vi "Init.vi"(5 "Overwrite Lib Path":path, 7 "ndim":i32, 8 "error in (no error)":errorcluster, 9 "flann_params":T1={"algorithm"=0, "checks"=0, "eps"=0.0, "sorted"=1, "max_neighbors"=-1, "cores"=0, "trees"=0, "leaf_max_size"=0, "branching"=0, "iterations"=0, "centers_init"=0, "cb_index"=0.0, "target_precision"=0.0, "build_weight"=0.0, "memory_weight"=0.0, "sample_fraction"=0.0, "table_number_"=0, "key_size_"=0, "multi_probe_level_"=0, "log_level"=0, "random_seed"=0} {"algorithm" items=["FLANN_INDEX_LINEAR"=0, "FLANN_INDEX_KDTREE"=1, "FLANN_INDEX_KMEANS"=2, "FLANN_INDEX_COMPOSITE"=3, "FLANN_INDEX_KDTREE_SINGLE"=4, "FLANN_INDEX_HIERARCHICAL"=5, "FLANN_INDEX_LSH"=6, "FLANN_INDEX_SAVED"=254, "FLANN_INDEX_AUTOTUNED"=255]; "centers_init" items=["FLANN_CENTERS_RANDOM", "FLANN_CENTERS_GONZALES", "FLANN_CENTERS_KMEANSPP", "FLANN_CENTERS_GROUPWISE"]; "log_level" items=["FLANN_LOG_NONE", "FLANN_LOG_FATAL", "FLANN_LOG_ERROR", "FLANN_LOG_WARN", "FLANN_LOG_INFO", "FLANN_LOG_DEBUG"]}, 10 "index_ptr":u64, 11 "KD Tree in":refnum<class "KD Tree.lvclass">) -> (0 "error out":errorcluster, 3 "KD Tree out":refnum<class "KD Tree.lvclass">)   [LabVIEW 2020, in "KD Tree.lvlib" / "KD Tree.lvclass"]
uses:
  KD Tree.lvclass
  flann/Flann Params.ctl
  KD Tree.lvclass/KD Tree.ctl
  KD Tree.lvlib
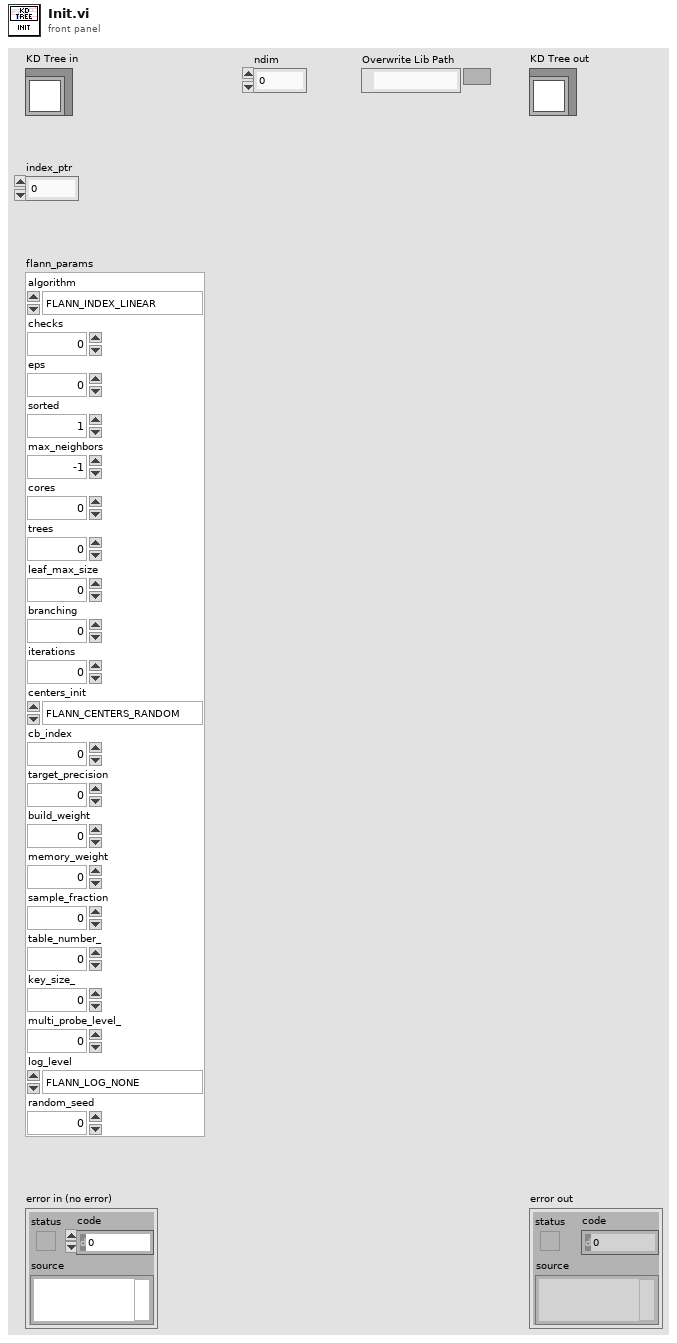
[diagram p1: front panel]
types:
  T1 = typedef "KD Tree.lvlib/Flann Params.ctl" = cluster{"algorithm":u32, "checks":i32, "eps":sgl, "sorted":i32, "max_neighbors":i32, "cores":i32, "trees":i32, "leaf_max_size":i32, "branching":i32, "iterations":i32, "centers_init":u32, "cb_index":sgl, "target_precision":sgl, "build_weight":sgl, "memory_weight":sgl, "sample_fraction":sgl, "table_number_":u32, "key_size_":u32, "multi_probe_level_":u32, "log_level":u32, "random_seed":i32}
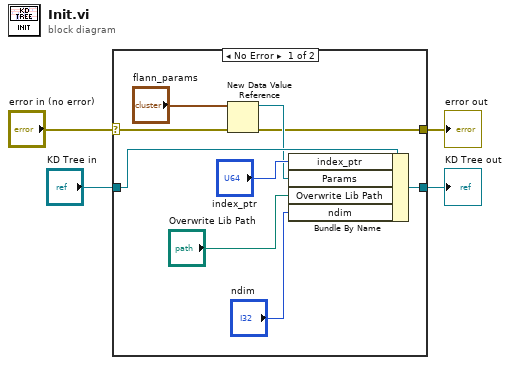
[diagram p0: block diagram]
diagram:
  n1 = case shown="No Error" "error in (no error)" {
    selector: "error in (no error)" -> [w12 w15]
    tunnel: [w5 w15] -> w3
    tunnel: [w11 w14] -> w1
    tunnel: "KD Tree in" -> [w13 w14]
    frame No Error {
      n2 = New Data Value Reference(data value="flann_params", error in=w12) -> (data value reference=w9:refnum<data-value>, error out=w5:errorcluster)
      n3 = Bundle By Name(cluster=w13, "index_ptr"="index_ptr", "Params"=w9, "Overwrite Lib Path"="Overwrite Lib Path", "ndim"="ndim") -> (w11:refnum<class "KD Tree.lvclass">)
    }
    frame Error {
    }
  }
  "error out" <- w3
  "KD Tree out" <- w1
